vi "AcquireWaveforms.vi"(8 "error in (no error)":errorcluster, 9 "Data Flow Maps":T2[](array[typedef]), 11 "923x Acquisition Config":T3={"NumberOfModules"=0, "Dynamic FPGA VI Ref"=refnum, "KeyphasorX3"=[], "FixedSizeX24"={"EnabledChannels"=[], "Sensitivity"=[], "InputConfig"=[]}, "SamplingInfo"={"Number of Channels"=4, "Sampling Rate"=4.0, "Channels"=[], "Units"=[]}, "BlockSize (sec)"=0.0, "Samples To Read (per chan)"=0, "RunningAcquisitionLength"=0.0, "Settling Time"=0.0, "Waveform Groups"=[], "Acquisition Block Number"=0, "Device Name"="", "ValidConfig"=FALSE} {"FixedSizeX24"."InputConfig" items=["AC Coupled", "DC Coupled", "IEPE AC Coupled"]}) -> (0 "error out":errorcluster, 1 "Data Flow Maps out":T2[](array[typedef]), 2 "Pulse Positions Array":T1[](array[typedef]), 3 "Waveforms":waveform(sgl)[](array[waveform]), 4 "log string":string, 5 "Data Rate [S/s]":u32, 6 "adjusted time":bool)   [LabVIEW 2015]
uses:
  <vilib>/addons/InsightCM/Devices/Shared/AcquireBaseLoop/controls/Configuration.ctl
  <vilib>/addons/InsightCM/Devices/Shared/AcquireBaseLoop/controls/TachometerConfig.ctl
  <vilib>/addons/InsightCM/Devices/Shared/AcquireBaseLoop/controls/FixedSizeArrays.ctl
  <vilib>/LabVIEW Targets/FPGA/cRIO/shared/nicrio_ModuleControls/nicrio_cRIO-9232_ConfigModeRing.ctl
  <vilib>/addons/InsightCM/Devices/Shared/cRIOWfmAcq/subVIs/RIO Wfm Cust Ctrls/rwfm_SamplingInfo.ctl
  <vilib>/addons/InsightCM/Devices/Shared/AcquireBaseLoop/controls/Group.ctl
  <vilib>/addons/InsightCM/Devices/Shared/AcquireBaseLoop/controls/Channel.ctl
  <vilib>/addons/InsightCM/Utilities/ChannelStatus/controls/RangeParams.ctl
  <vilib>/addons/PointValueMap/controls/PointMap.ctl
  <vilib>/addons/InsightCM/Utilities/Analysis/Shared/controls/PulsePositions.ctl
  <vilib>/addons/PointValueMap/PointValueMap.lvlib
  <vilib>/addons/PointValueMap/subVIs/Point_Write_double.vi
  <vilib>/addons/InsightCM/Devices/Shared/AcquireBaseLoop/FpgaAcquisition923x.lvlib
  <vilib>/addons/InsightCM/Devices/Shared/cRIOWfmAcq/cRIOWfmLib.lvlib
  <vilib>/addons/InsightCM/Utilities/Analysis/Shared/AnalysisHelper.lvlib
  <vilib>/addons/InsightCM/Utilities/ChannelStatus/ChannelStatus.lvlib
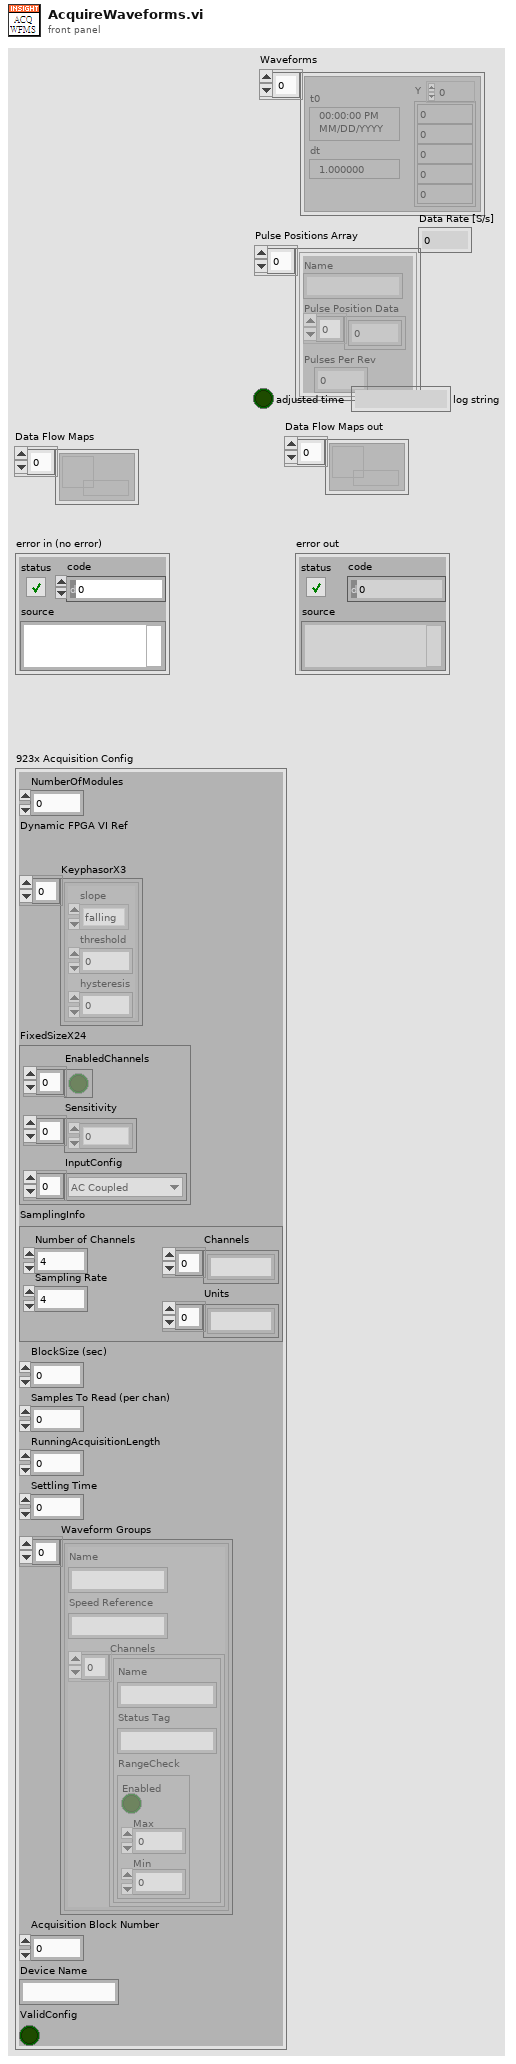
[diagram p1: front panel]
types:
  T1 = typedef "AnalysisHelper.lvlib/PulsePositions.ctl" = cluster{"Name":string, "Pulse Position Data":dbl[], "Pulses Per Rev":i32}
  T2 = typedef "PointValueMap.lvlib/PointMap.ctl" = refnum<data-value>
  T3 = typedef "FpgaAcquisition923x.lvlib/Configuration.ctl" = cluster{"NumberOfModules":i16, "Dynamic FPGA VI Ref":refnum<k20>, "KeyphasorX3":T4[], "FixedSizeX24":T5, "SamplingInfo":T7, "BlockSize (sec)":dbl, "Samples To Read (per chan)":i32, "RunningAcquisitionLength":dbl, "Settling Time":dbl, "Waveform Groups":T8[], "Acquisition Block Number":i32, "Device Name":string, "ValidConfig":bool}
  T4 = typedef "FpgaAcquisition923x.lvlib/TachometerConfig.ctl" = cluster{"slope":enum16{"falling", "rising"}, "threshold":dbl, "hysteresis":dbl}
  T5 = typedef "FpgaAcquisition923x.lvlib/FixedSizeArrays.ctl" = cluster{"EnabledChannels":bool[], "Sensitivity":dbl[], "InputConfig":T6[]}
  T6 = typedef "nicrio_cRIO-9232_ConfigModeRing.ctl" = u8
  T7 = typedef "cRIOWfmLib.lvlib/rwfm_SamplingInfo.ctl" = cluster{"Number of Channels":i32, "Sampling Rate":dbl, "Channels":string[], "Units":string[]}
  T8 = typedef "FpgaAcquisition923x.lvlib/Group.ctl" = cluster{"Name":string, "Speed Reference":string, "Channels":T9[]}
  T9 = typedef "FpgaAcquisition923x.lvlib/Channel.ctl" = cluster{"Name":string, "Status Tag":string, "RangeCheck":T10}
  T10 = typedef "ChannelStatus.lvlib/RangeParams.ctl" = cluster{"Enabled":bool, "Max":dbl, "Min":dbl}
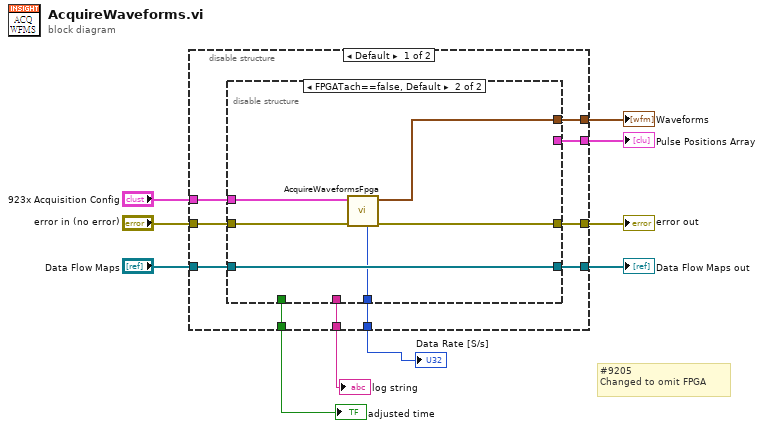
[diagram p0: block diagram]
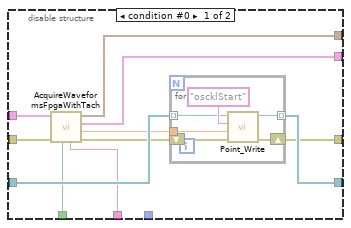
[diagram p2: hidden frame]
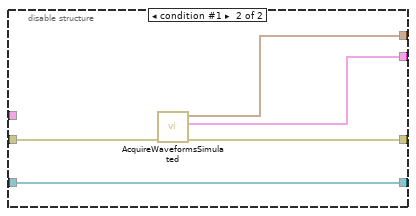
[diagram p3: hidden frame]
diagram:
  # "#9205\nChanged to omit FPGA"
  n1 = disable-structure shown="Default" {
    disable-tunnel: "error in (no error)" -> [w20 w48]
    disable-tunnel: [w19 w47] -> w8
    disable-tunnel: [w18 w46] -> w5
    disable-tunnel: [w17 w45] -> w7
    disable-tunnel: "Data Flow Maps" -> [w16 w44]
    disable-tunnel: [w15 w44] -> w10
    disable-tunnel: "923x Acquisition Config" -> [w14 _]
    disable-tunnel: [w13 _] -> w3
    disable-tunnel: [w12 _] -> w2
    disable-tunnel: [w11 _] -> w1
    frame condition #0 (active) {
      n2 = disable-structure shown="FPGATach==false, Default" {
        disable-tunnel: w20 -> [w30 w43]
        disable-tunnel: [w23 w42] -> w18
        disable-tunnel: [w31 w41] -> w19
        disable-tunnel: [w29 _] -> w17
        disable-tunnel: w16 -> [w28 w40]
        disable-tunnel: [w26 w40] -> w15
        disable-tunnel: w14 -> [w25 w39]
        disable-tunnel: [w22 _] -> w13
        disable-tunnel: [w21 _] -> w12
        disable-tunnel: [_ w38] -> w11
        frame condition #0 {
          n3 = call <vilib>:"AcquireWaveformsFpgaWithTach.vi"("error in (no error)"=w30, "923x Acquisition Config"=w25) -> ("error out"=w24:errorcluster, "OSClkStart"=w27:dbl, "Pulse Positions Array"=w29:T1[], "Waveforms"=w31:waveform(sgl)[], "log string"=w21:string, "adjusted time"=w22:bool)  [unwired: 4 in]
          n4 = for {
            tunnel: w28 -> [w36] mode=indexing
            tunnel: w27 -> [w35]
            tunnel: [w33] -> w26 mode=indexing
            shift-right: [w32] -> w23
            shift-left: w24 -> [w34]
            n5 = call-poly <vilib>:"Point_Write.vi"("Error In"=w34, "Value"=w35, "Tag"="oscklStart", "Map"=w36) -> ("Error Out"=w32:errorcluster, "Map Out"=w33:T2)  [unwired: 6 in]
          }
        }
        frame condition #1 (active) {
          n6 = call "AcquireWaveformsFpga.vi"("error in (no error)"=w43, "923x Acquisition Config"=w39) -> ("error out"=w42:errorcluster, "Waveforms"=w41:waveform(sgl)[], "Data Rate [S/s]"=w38:u32)  [unwired: 7 in]
        }
      }
    }
    frame condition #1 {
      n7 = call <vilib>:"AcquireWaveformsSimulated.vi"("error in (no error)"=w48) -> ("error out"=w46:errorcluster, "simulated pulse position array"=w45:T1[], "simulated waveforms"=w47:waveform(sgl)[])  [unwired: 8 in]
    }
  }
  "error out" <- w5
  "Data Flow Maps out" <- w10
  "Waveforms" <- w8
  "Pulse Positions Array" <- w7
  "adjusted time" <- w3
  "log string" <- w2
  "Data Rate [S/s]" <- w1
